vi "Pre-Actor.vi"(8 "error in (no error)":errorcluster, 11 "Main in":refnum<class "Main.lvclass">) -> (0 "error out":errorcluster, 3 "Main out":refnum<class "Main.lvclass">)   [LabVIEW 2023, in "Main.lvlib" / "Main.lvclass"]
doc: "<b>Pre-Actor </b>\nThis routine is called before registering for events, after control references have been mapped to the class private data. It is inteded to perform any additional actions before the actor front panel is displayed.\n\n<b>Main</b>\nAt the main level, this routine links the splitter references which is unique to the main UI, applies branding logos, then launches the subordinate classes:\n1. Fault Monitor\n2. Right Manual Buttons (hidden)\n3. ManualUI (hidden)\n4. Future items:\n a. Configuration Editor (prime panel - Hidden)\n b. Report Viewer (prime panel - Hidden)"
uses:
  Library/Main.lvclass
  Library/Main.lvclass/Main.ctl
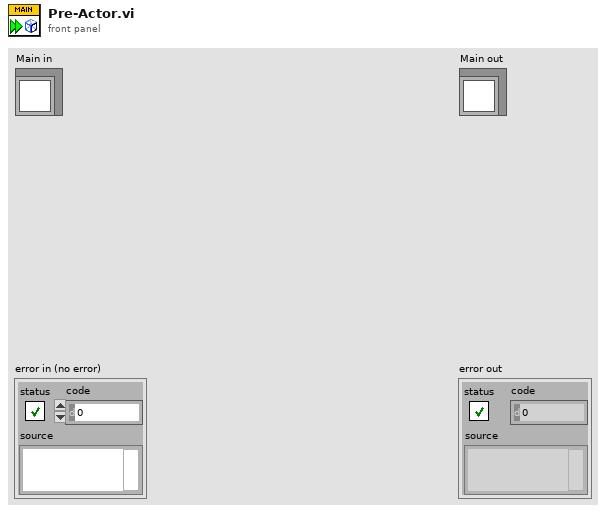
[diagram p1: front panel]
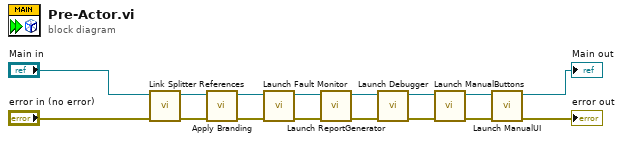
[diagram p0: block diagram]
diagram:
  n1 = call "Link Splitter References.vi"("error in (no error)"="error in (no error)", "Main in"="Main in") -> ("error out"=w13:errorcluster, "Main out"=w14:refnum<class "Main.lvclass">)  [unwired: 8 in]
  n2 = call "Apply Branding.vi"("error in (no error)"=w13, "Main in"=w14) -> ("error out"=w11:errorcluster, "Main out"=w12:refnum<class "Main.lvclass">)  [unwired: 8 in]
  n3 = call "Launch Fault Monitor.vi"("error in (no error)"=w11, "Main in"=w12) -> ("error out"=w3:errorcluster, "Main out"=w4:refnum<class "Main.lvclass">)  [unwired: 8 in]
  n4 = call "Launch ReportGenerator.vi"("error in (no error)"=w3, "Main in"=w4) -> ("error out"=w1:errorcluster, "Main out"=w2:refnum<class "Main.lvclass">)  [unwired: 8 in]
  n5 = call "Launch Debugger.vi"("error in (no error)"=w1, "Main in"=w2) -> ("error out"=w9:errorcluster, "Main out"=w10:refnum<class "Main.lvclass">)  [unwired: 8 in]
  n6 = call "Launch ManualButtons.vi"("error in (no error)"=w9, "Main in"=w10) -> ("error out"=w7:errorcluster, "Main out"=w8:refnum<class "Main.lvclass">)  [unwired: 8 in]
  n7 = call "Launch ManualUI.vi"("error in (no error)"=w7, "Main in"=w8) -> ("error out"=→"error out":errorcluster, "Main out"=→"Main out":refnum<class "Main.lvclass">)  [unwired: 8 in]
